vi "graph-teste.vi"() -> ()   [LabVIEW 2014]
panel:
  in  "length":i32=100
  in  "index":i32=96
  out "XY Graph 2":cluster{dbl[], dbl[]}(graph)={[96.0, 97.0, 98.0, 99.0, 100.0, 101.0, 102.0, 103.0, 104.0, 105.0, 106.0, 107.0, 108.0, 109.0, 110.0, 111.0, 112.0, 113.0, 114.0, 115.0, 116.0, 117.0, 118.0, 119.0, 120.0, 121.0, 122.0, 123.0, 124.0, 125.0, 126.0, 127.0, 128.0, 129.0, 130.0, 131.0, 132.0, 133.0, 134.0, 135.0, 136.0, 137.0, 138.0, 139.0, 140.0, 141.0, 142.0, 143.0, 144.0, 145.0, 146.0, 147.0, 148.0, 149.0, 150.0, 151.0, 152.0, 153.0, 154.0, 155.0, 156.0, 157.0, 158.0, 159.0, 160.0, 161.0, 162.0, 163.0, 164.0, 165.0, 166.0, 167.0, 168.0, 169.0, 170.0, 171.0, 172.0, 173.0, 174.0, 175.0, 176.0, 177.0, 178.0, 179.0, 180.0, 181.0, 182.0, 183.0, 184.0, 185.0, 186.0, 187.0, 188.0, 189.0, 190.0, 191.0, 192.0, 193.0, 194.0, 195.0], [0.000113759649, 0.000124082972, 0.000160865863, 0.000232850685, 0.000221431974, 0.00020880972, 0.000182131541, 0.000189555321, 0.00018384365, 0.000201535525, 0.000222851828, 0.000238442672, 0.000250618496, 0.000298449575, 0.000393660722, 0.000422396199, 0.000472178746, 0.000469877505, 0.000483084269, 0.000541319247, 0.000523638864, 0.000606568323, 0.000696857114, 0.000801942855, 0.000827191958, 0.000925799736, 0.001010503466, 0.001022713805, 0.001151157032, 0.001220405675, 0.001203233885, 0.001201721983, 0.001426163355, 0.001475591525, 0.001532070659, 0.001513541134, 0.001506131161, 0.00169205915, 0.001848151685, 0.001978981283, 0.002024893139, 0.002138007868, 0.002232954384, 0.002232864632, 0.002245295881, 0.002390867169, 0.002540829221, 0.002693720744, 0.002598461248, 0.002722872715, 0.002789960543, 0.002988117254, 0.00304582525, 0.003184140697, 0.003369286333, 0.00348535354, 0.003292457408, 0.003554947341, 0.003709626939, 0.003737734177, 0.003895262656, 0.003762548361, 0.003928476321, 0.004042631178, 0.003974033813, 0.004213184672, 0.004262396516, 0.004286651513, 0.00444728673, 0.004390091886, 0.004537094664, 0.004577391567, 0.004643568112, 0.004513410367, 0.004888361627, 0.004865984465, 0.00498832257, 0.004972082735, 0.005164090517, 0.005265528825, 0.005316864713, 0.005231203702, 0.005251304931, 0.005242067794, 0.004914522026, 0.005222937669, 0.005252671829, 0.005249878168, 0.005077589555, 0.005152393426, 0.005165374624, 0.00509835586, 0.005639955285, 0.005516547183, 0.005219665272, 0.005271081696, 0.00567516874, 0.005639474336, 0.005683802971, 0.005508762058]}
  out "XY Graph":cluster{dbl[], dbl[]}(graph)
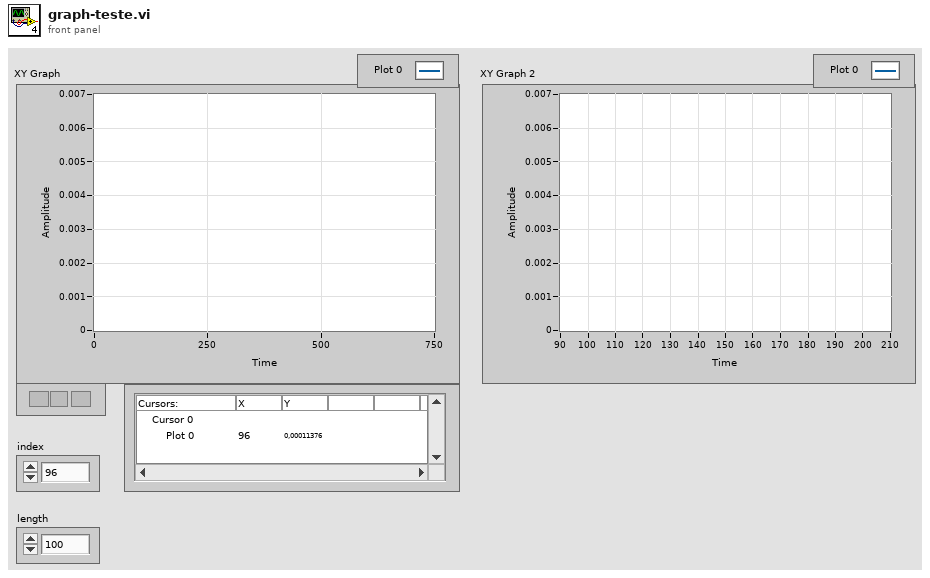
[diagram p1: front panel]
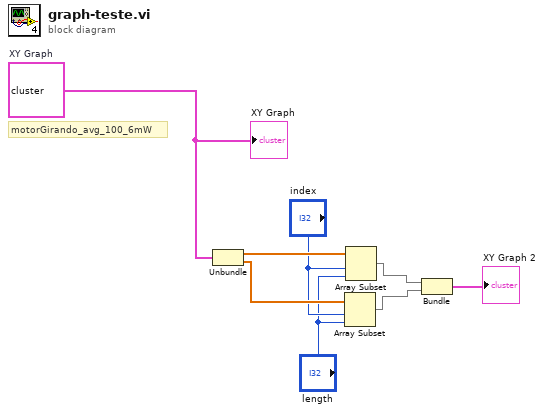
[diagram p0: block diagram]
diagram:
  w8 = cluster{dbl[], dbl[]} {array[716 elements], array[716 elements]}  # XY Graph
  # "motorGirando_avg_100_6mW"
  n1 = Unbundle(w8) -> (w7:dbl[], w6:dbl[])
  n2 = Array Subset(array=w6, index="index", length="length") -> (w1:dbl[])
  n3 = Array Subset(array=w7, index="index", length="length") -> (w5:dbl[])
  n4 = Bundle(w5, w1) -> (→"XY Graph 2":cluster{dbl[], dbl[]})  [unwired: 1 in]
  "XY Graph" <- w8
